vi "write data cell with column offset.vi"(5 "Column relative?":bool, 6 "Data Input":dbl, 7 "data column":i32=6, 8 "error in (no error)":errorcluster, 9 "row offset":i32, 10 "start of last occupied row":cluster{"row":i32, "column":i32}, 11 "NI_report in":refnum<class "NI_report.lvclass">) -> (0 "error out":errorcluster, 3 "NI_report out":refnum<class "NI_report.lvclass">)   [LabVIEW 2016]
uses:
  <vilib>/Utility/NIReport.llb/NI_report.lvclass
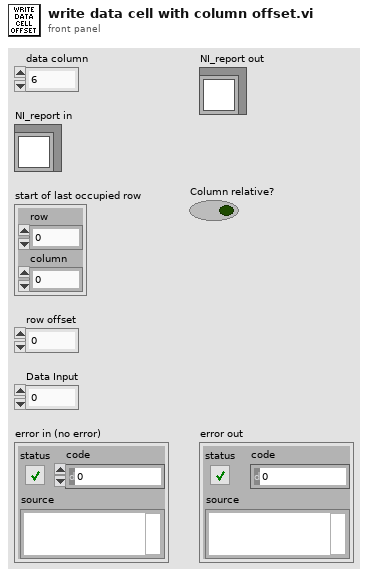
[diagram p1: front panel]
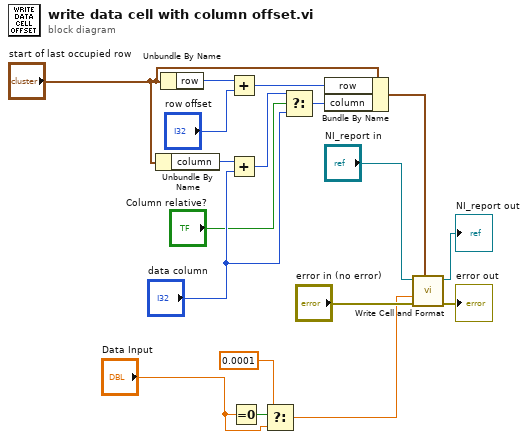
[diagram p0: block diagram]
diagram:
  n1 = Unbundle By Name("start of last occupied row") -> ("column"=w9:i32)
  n2 = Unbundle By Name("start of last occupied row") -> ("row"=w10:i32)
  n3 = Add(x=w10, y="row offset") -> (x+y=w14:i32)
  n4 = Add(x=w9, y="data column") -> (x+y=w7:i32)
  n5 = Equal To 0?(x="Data Input") -> (x = 0?=w4:bool)
  n6 = Select(t=0.0001, s=w4, f="Data Input") -> (s? t:f=w2:dbl)
  n7 = Select(t=w7, s="Column relative?", f="data column") -> (s? t:f=w8:i32)
  n8 = Bundle By Name(cluster="start of last occupied row", "row"=w14, "column"=w8) -> (w15:cluster{"row":i32, "column":i32})
  n9 = call "Write Cell and Format.vi"("output cluster"=w15, "error in (no error)"="error in (no error)", "Data In"=w2, "NI_report in"="NI_report in") -> ("error out"=→"error out":errorcluster, "NI_report out"=→"NI_report out":refnum<class "NI_report.lvclass">)  [unwired: 6 in]
